vi "LSMcontroller_v64_updatedwaveformhandling.vi"() -> ()   [LabVIEW 2015] (continued)
                                n91 = local write "# of frames"(1 ("# of frames")) -> ()
                                }
                                }
                                }
                                }
                              }
                            }
                          }
                        }
                        n92 = local write "ROI Type"(w2086) -> ()
                      }
                      frame #1 {
                        # "change active waveform numbers array"
                        n93 = local read "save\ndata"() -> (w2126:bool)
                        n94 = Get Date/Time In Seconds() -> (seconds since 1Jan1904=w2128:timestamp)
                        n95 = case shown="True" w2126 {
                          tunnel: w2128 -> [w2129 w2131]
                          tunnel: [w2129 w2130] -> w2127
                          frame False {
                          }
                          frame True {
                            n96 = call "createdatafolder.vi"("timestamp in"=w2131) -> ("current data path"=w2132:path, "timestamp out"=w2130:timestamp)
                            n97 = local write "data dir"(w2132) -> ()
                          }
                        }
                        n98 = stacked-sequence {
                          tunnel: w2127 -> [_ w2139 _ _ _ _ _ _ _ _]
                          tunnel: [_ _ _ _ _ w2282 _ _ _ _] -> w2125
                          tunnel: [_ _ _ _ _ w2281 _ _ _ _] -> w2124
                          tunnel: [_ _ _ _ _ w2280 _ _ _ _] -> w2123
                          tunnel: [_ _ _ _ _ w2279 _ _ _ _] -> w2122
                          tunnel: [_ _ _ _ _ w2278 _ _ _ _] -> w2121
                          tunnel: [_ _ _ _ _ w2277 _ _ _ _] -> w2120
                          tunnel: [_ _ _ _ _ w2276 _ _ _ _] -> w2119
                          tunnel: [_ _ _ _ _ w2275 _ _ _ _] -> w2118
                          tunnel: [_ _ _ _ _ w2274 _ _ _ _] -> w2117
                          tunnel: [_ _ _ _ _ w2273 _ _ _ _] -> w2116
                          tunnel: [_ _ _ _ _ w2272 _ _ _ _] -> w2115
                          tunnel: [_ _ _ _ _ w2271 _ _ _ _] -> w2114
                          tunnel: [_ _ _ _ _ w2270 _ _ _ _] -> w2113
                          tunnel: [_ _ _ _ _ w2269 _ _ _ _] -> w2112
                          frame #0 {
                            n99 = local read "AI channels"() -> (w2138:i32[])
                            n100 = local read "CI channels"() -> (w2137:i32[])
                            n101 = call "2pparameters.vi"("command"="get") -> ("params out"=w2135:T10)  [unwired: 1 in]
                            n102 = Bundle By Name(cluster=w2135, "aAI"=w2138, "aCI"=w2137) -> (w2136:T10)
                            n103 = call "2pparameters.vi"("Params in"=w2136, "command"="set") -> ()  [unwired: 1 out]
                          }
                          frame #1 {
                            n104 = local read "Vy-min ref"() -> (w2143:dbl)
                            n105 = local read "Vy-max ref"() -> (w2144:dbl)
                            n106 = local read "Angle ref"() -> (w2142:dbl)
                            n107 = local read "Vx-min ref"() -> (w2145:dbl)
                            n108 = local write "counts"(0 ("counts")) -> ()
                            n109 = local write "graphtab"(T5."image" ("graphtab")) -> ()
                            n110 = local read "Vx-max ref"() -> (w2146:dbl)
                            n111 = property on="Stop" class="Bool (strict)"("Visible"=TRUE, "DisabledEnum"=T7."Enabled" ("Disabled")) -> ()  [unwired: 2 in, 2 out]
                            n112 = property on="Start" class="Bool (strict)"("Visible"=FALSE, "DisabledEnum"=T7."Disabled and Grayed Out" ("Disabled")) -> ()  [unwired: 2 in, 2 out]
                            n113 = script code="Xic=(ximax+ximin)./2;\nYic=(yimax+yimin)./2;\nximin=ximin-Xic;\nymin=ymin-Yic;\nxirmin=ximin.*cos(pi/180.*phi)+yimin.*sin(pi./180.*phi)+Xic;\nyirmin=-ximin.*sin(pi./180.*phi)+yimin.*cos(pi./180.*phi)+Yic;"("ximax"=w2146, "ximin"=w2145, "yimax"=w2144, "yimin"=w2143, "phi"=w2142) -> ("xirmin"=w2141:dbl, "yirmin"=w2140:dbl)  [unwired: 1 in, 1 out]
                            n114 = stacked-sequence {
                              tunnel: w2139 -> [_ w2171 _]
                              frame #0 {
                                n115 = local read "Measurement"() -> (w2153:T4)
                                n116 = case shown="\"X-Y-Z stack\"" w2153 {
                                frame "X-Y-t movie", Default {
                                n117 = call "2pparameters.vi"("command"="get") -> ("params out"=w2156:T10)  [unwired: 1 in]
                                n118 = Bundle By Name(cluster=w2156, "type"="X-Y-t movie") -> (w2154:T10)
                                n119 = call "2pparameters.vi"("Params in"=w2154, "command"="set") -> ()  [unwired: 1 out]
                                }
                                frame "X-Y-Z stack" {
                                n120 = call "2pparameters.vi"("command"="get") -> ("params out"=w2161:T10)  [unwired: 1 in]
                                n121 = Bundle By Name(cluster=w2161, "type"="X-Y-Z stack") -> (w2159:T10)
                                n122 = call "2pparameters.vi"("Params in"=w2159, "command"="set") -> ()  [unwired: 1 out]
                                }
                                frame "Lifetime (scan)" {
                                n123 = call "2pparameters.vi"("command"="get") -> ("params out"=w2166:T10)  [unwired: 1 in]
                                n124 = Bundle By Name(cluster=w2166, "type"="Lifetime (scan)") -> (w2164:T10)
                                n125 = call "2pparameters.vi"("Params in"=w2164, "command"="set") -> ()  [unwired: 1 out]
                                }
                                }
                              }
                              frame #1 {
                                n126 = Format Date/Time String(time format string (%c)="%Y%m%d", seconds (now)=w2171) -> (date/time string=w2170:string)  [unwired: 1 in]
                                n127 = Format Date/Time String(time format string (%c)="%H%M%S", seconds (now)=w2171) -> (date/time string=w2169:string)  [unwired: 1 in]
                                n128 = call "2pparameters.vi"("command"="get") -> ("params out"=w2175:T10)  [unwired: 1 in]
                                n129 = Bundle By Name(cluster=w2175, "date"=w2170, "time"=w2169) -> (w2174:T10)
                                n130 = call "2pparameters.vi"("Params in"=w2174, "command"="set") -> ()  [unwired: 1 out]
                              }
                              frame #2 {
                                n131 = call "configuration.vi"("command"="get") -> ("config out"=w2185:T11)  [unwired: 2 in, 1 out]
                                n132 = Unbundle By Name(w2185) -> ("CI names"=w2186:string[], "AI names"=w2187:string[])
                                n133 = call "2pparameters.vi"("command"="get") -> ("params out"=w2181:T10)  [unwired: 1 in]
                                n134 = Unbundle By Name(w2181) -> ("aCI"=w2182:i32[], "aAI"=w2183:i32[])
                                n135 = for {
                                tunnel: w2182 -> [w2197] mode=indexing
                                tunnel: w2186 -> [w2198]
                                tunnel: [w2196] -> w2188 mode=indexing
                                n136 = Index Array(array=w2198, index=w2197) -> (element=w2196:string)
                                }
                                n137 = for {
                                tunnel: w2183 -> [w2194] mode=indexing
                                tunnel: w2187 -> [w2195]
                                tunnel: [w2193] -> w2189 mode=indexing
                                n138 = Index Array(array=w2195, index=w2194) -> (element=w2193:string)
                                }
                                n139 = Build Array (concatenate)(w2188, w2189) -> (w2179:string[])
                                n140 = for {
                                tunnel: w2179 -> [w2191] mode=indexing
                                tunnel: [w2190] -> w2178 mode=indexing
                                i -> [w2192]
                                n141 = Bundle("String"=w2191, w2192) -> (w2190:cluster{"String":string, i32})  [unwired: 1 in]
                                }
                                n142 = property on="image1list" class="Ring (strict)"("StringsAndValues[]"=w2178) -> ()  [unwired: 2 in, 2 out]
                                n143 = property on="image2list" class="Ring (strict)"("StringsAndValues[]"=w2178) -> ()  [unwired: 2 in, 2 out]
                              }
                            }
                            n144 = call "setposition.vi"("Vy"=w2140, "Vx"=w2141) -> ()  [unwired: 1 in]
                          }
                          frame #2 {
                            n145 = call "X-array-databuffer.vi"("command"=enum16{"get", "set", "clear", "append"}."clear") -> ()  [unwired: 3 in, 2 out]
                            n146 = call "Y-array-databuffer.vi"("command"=enum16{"get", "set", "clear", "append"}."clear") -> ()  [unwired: 3 in, 2 out]
                            n147 = call "2pparameters.vi"("command"="get") -> ("params out"=w2201:T10)  [unwired: 1 in]
                            n148 = Unbundle By Name(w2201) -> ("autoshutter"=w2202:bool, "auto OD"=w2199:bool)
                            n149 = call "allAI-temp_img.vi"("command"=enum16{"get", "set", "clear", "append"}."clear") -> ()  [unwired: 3 in, 2 out]
                            n150 = case shown="True" w2199 {
                              frame False {
                              }
                              frame True {
                                n151 = call "configuration.vi"("command"="get") -> ("config out"=w2210:T11)  [unwired: 2 in, 1 out]
                                n152 = Unbundle By Name(w2210) -> ("image OD"=w2211:u16)
                                n153 = local read "ODfilt"() -> (w2208:u16)
                                n154 = call "filterwheelcontrol_nothorlabslib.vi"("Current OD filt"=w2208, "New ODfilt"=w2211) -> ()  [unwired: 1 in]
                              }
                            }
                            n155 = case shown="True" w2202 {
                              frame False {
                              }
                              frame True {
                                n156 = call "shuttercontrol.vi"("command"="close") -> ()  [unwired: 1 in, 1 out]
                              }
                            }
                            n157 = call "CH1-temp.vi"("command"=enum16{"get", "set", "clear", "add row"}."clear") -> ()  [unwired: 3 in, 2 out]
                            n158 = call "CH2-temp.vi"("command"=enum16{"get", "set", "clear", "add row"}."clear") -> ()  [unwired: 3 in, 2 out]
                          }
                          frame #3 {
                            n159 = local read "avpp"() -> (w2245:i32)
                            n160 = local read "Angle ref"() -> (w2244:dbl)
                            n161 = local read "ROI Type"() -> (w2243:u16)
                            n162 = local read "xpixels ref"() -> (w2240:i32)
                            n163 = local read "Vx-min ref"() -> (w2239:dbl)
                            n164 = local read "Vx-max ref"() -> (w2238:dbl)
                            n165 = local read "ypixels ref"() -> (w2236:i32)
                            n166 = local read "Vy-min ref"() -> (w2237:dbl)
                            n167 = local read "Vy-max ref"() -> (w2233:dbl)
                            n168 = local read "Sampling rate"() -> (w2227:dbl)
                            n169 = local read "finite samples"() -> (w2228:bool)
                            n170 = local read "continuous"() -> (w2231:bool)
                            n171 = local read "wavdet"() -> (w2232:bool)
                            n172 = local read "# of frames"() -> (w2230:i32)
                            n173 = local read "maxbufferAI"() -> (w2229:i32)
                            n174 = local read "Override AI buffer"() -> (w2213:bool)
                            n175 = call "2pparameters.vi"("command"="get") -> ("params out"=w2242:T10)  [unwired: 1 in]
                            n176 = Bundle By Name(cluster=w2242, "avpp"=w2245, "Angle Img"=w2244, "Xpixels Img"=w2240, "Vx-min Img"=w2239, "VX-max Img"=w2238, "Ypixels Img"=w2236, "Vy-min Img"=w2237, "Vy-max Img"=w2233, "srate"=w2227, "srate Img"=w2227, "finite"=w2228, "cont"=w2231, "wavdet"=w2232, "measpoints"=w2230, "maxbufferAI"=w2229, "Drawing Mode"=w2243, "Vz-reset"=0.0, "AIoverride"=w2213) -> (w2234:T10)
                            n177 = call "2pparameters.vi"("Params in"=w2234, "command"="set") -> ()  [unwired: 1 out]
                            n178 = local read "Vholding (mV)"() -> (w2216:sgl)
                            n179 = local read "Current Clamp"() -> (w2222:bool)
                            n180 = local read "Voltage Clamp"() -> (w2221:bool)
                            n181 = local read "OCgain"() -> (w2217:sgl)
                            n182 = local read "CC_ICgain"() -> (w2220:dbl)
                            n183 = local read "holdon"() -> (w2215:bool)
                            n184 = call "patchparameters.vi"("command"="get") -> ("Params out"=w2224:T13)  [unwired: 1 in]
                            n185 = Bundle By Name(cluster=w2224, "VC"=w2221, "CC"=w2222, "CC_icg (pA/mv)"=w2220, "VC_icg (mV/mV)"=sgl 10.0, "OCG (mV/pA)"=w2217, "OVG (mV/mV)"=0.1, "Vhold (mV)"=w2216, "holdon"=w2215) -> (w2223:T13)
                            n186 = call "patchparameters.vi"("Params in"=w2223, "command"="set") -> ()  [unwired: 1 out]
                          }
                          frame #4 {
                            # "Generate Waveforms for Scanning Mirrors"
                            n187 = call "2pparameters.vi"("command"="get") -> ("params out"=w2260:T10)  [unwired: 1 in]
                            n188 = Unbundle By Name(w2260) -> ("srate Img"=w2259:sgl, "Angle Img"=w2258:dbl, "VX-max Img"=w2257:dbl, "Vx-min Img"=w2256:dbl, "Xpixels Img"=w2255:i32, "Ypixels Img"=w2254:i32, "Vy-max Img"=w2253:dbl, "Vy-min Img"=w2252:dbl, "Drawing Mode"=w2251:u16)
                            n189 = call "ROI-databuffer.vi"("command"=enum16{"get", "set", "clear", "append"}."get") -> ("array out"=w2250:cluster{"x":sgl, "y":sgl}[])  [unwired: 4 in]
                            n190 = call "ScanningWaveform_v4.vi"("Vy-min"=w2252, "Vy-max"=w2253, "yPixels/tPixels"=w2254, "xPixels/rPixels"=w2255, "Vx-min"=w2256, "Vx-max"=w2257, "Drawing Mode"=w2251, "Angle"=w2258, "AOrate"=w2259, "Points"=w2250) -> ("numPixels"=w2246:dbl, "Y-WaveArray"=w2249:dbl[], "P"=w2247:dbl, "X-WaveArray"=w2248:dbl[])  [unwired: 6 in]
                            n191 = call "2pparameters.vi"("command"="get") -> ("params out"=w2268:T10)  [unwired: 1 in]
                            n192 = call "Y-array-databuffer.vi"("array in"=w2249, "command"=enum16{"get", "set", "clear", "append"}."set") -> ()  [unwired: 2 in, 2 out]
                            n193 = call "X-array-databuffer.vi"("array in"=w2248, "command"=enum16{"get", "set", "clear", "append"}."set") -> ()  [unwired: 2 in, 2 out]
                            n194 = Bundle By Name(cluster=w2268, "P"=w2247, "sAOxy"=w2246) -> (w2265:T10)
                            n195 = call "2pparameters.vi"("Params in"=w2265, "command"="set") -> ()  [unwired: 1 out]
                          }
                          frame #5 {
                            # "rem2Ps"
                            # "A2Ps"
                            # "Al"
                            # "Rl"
                            n196 = stacked-sequence {
                              seq-local: [w2287 _ _ _ _ _ _ _ _ _ _] -> [_ w2399 _ w2454 _ w2534 _ _ _ _ _]
                              seq-local: [w2288 _ _ _ _ _ _ _ _ _ _] -> [_ w2400 w2410 _ w2503 _ _ _ _ _ _]
                              seq-local: [_ _ w2409 _ _ _ _ _ _ _ _] -> [_ _ _ _ w2497 _ _ _ _ _ _]
                              seq-local: [_ _ _ w2453 _ _ _ _ _ _ _] -> [_ _ _ _ _ w2533 _ _ _ _ _]
                              seq-local: [w2284 _ _ _ _ _ _ _ _ _ _] -> [_ w2396 _ _ _ _ _ _ w2719 w2787 _]
                              seq-local: [w2283 _ _ _ _ _ _ _ _ _ _] -> [_ w2395 _ _ _ _ _ _ w2720 w2788 _]
                              seq-local: [w2290 _ _ _ _ _ _ _ _ _ _] -> [_ _ _ _ _ _ w2572 _ w2718 w2786 _]
                              seq-local: [w2286 _ _ _ _ _ _ _ _ _ _] -> [_ w2394 _ _ _ _ w2571 w2639 _ _ _]
                              seq-local: [w2285 _ _ _ _ _ _ _ _ _ _] -> [_ w2393 _ _ _ _ w2570 w2638 _ _ _]
                              seq-local: [w2289 _ _ _ _ _ _ _ _ _ _] -> [_ _ _ _ _ _ w2569 w2637 _ _ _]
                              tunnel: [_ _ w2408 _ _ _ _ _ _ _ _] -> w2281
                              tunnel: [_ _ w2407 _ _ _ _ _ _ _ _] -> w2280
                              tunnel: [w2288 _ _ _ _ _ _ _ _ _ _] -> w2282
                              tunnel: [w2287 _ _ _ _ _ _ _ _ _ _] -> w2279
                              tunnel: [_ _ _ w2452 _ _ _ _ _ _ _] -> w2278
                              tunnel: [_ _ _ w2451 _ _ _ _ _ _ _] -> w2277
                              tunnel: [w2286 _ _ _ _ _ _ _ _ _ _] -> w2276
                              tunnel: [w2285 _ _ _ _ _ _ _ _ _ _] -> w2275
                              tunnel: [_ _ _ _ _ _ w2568 _ _ _ _] -> w2274
                              tunnel: [_ _ _ _ _ _ _ w2636 _ _ _] -> w2273
                              tunnel: [w2284 _ _ _ _ _ _ _ _ _ _] -> w2272
                              tunnel: [w2283 _ _ _ _ _ _ _ _ _ _] -> w2271
                              tunnel: [_ _ _ _ _ _ _ _ w2717 _ _] -> w2270
                              tunnel: [_ _ _ _ _ _ _ _ _ w2785 _] -> w2269
                              frame #0 {
                                # "for a next version, give ome thought to\nthe possibilit of intermittently updating the\nwaveforms. it will have to be a calculation\nbased on speed of CPU and program on the one hand\nand length of measurement on the other. but then it should be possible, in principle, to \nupdate the waveform on the fly and that way cut up a longer measurement in smaller parts."
                                # "Y"
                                # "X"
                                n197 = stacked-sequence {
                                tunnel: [w2291 _ _ _] -> w2288
                                tunnel: [_ w2303 _ _] -> w2287
                                tunnel: [_ _ _ w2360] -> w2283
                                tunnel: [_ _ _ w2359] -> w2284
                                tunnel: [_ _ _ w2358] -> w2290
                                tunnel: [_ _ w2318 _] -> w2286
                                tunnel: [_ _ w2317 _] -> w2285
                                tunnel: [_ _ w2316 _] -> w2289
                                frame #0 {
                                n198 = call "configuration.vi"("command"="get") -> ("config out"=w2293:T11)  [unwired: 2 in, 1 out]
                                n199 = Unbundle By Name(w2293) -> ("Voltage to Xgalvo"=w2292:i32)
                                n200 = call "2pparameters.vi"("command"="get") -> ("params out"=w2297:T10)  [unwired: 1 in]
                                n201 = in-place {
                                in-place-border: w2292 -> [w2302]
                                in-place-border: [w2299] -> w2291
                                n202 = in-place-cluster #1(w2297) -> ("aAO"=w2301:u32[])
                                n203 = call "add channel to active arrayv2.vi"("line array in"=w2301, "line to add"=w2302) -> ("line array out"=w2300:u32[], "addition"=w2299:bool)  [unwired: 1 out]
                                n204 = in-place-cluster #1("aAO"=w2300) -> (w2295:T10)
                                }
                                n205 = call "2pparameters.vi"("Params in"=w2295, "command"="set") -> ()  [unwired: 1 out]
                                }
                                frame #1 {
                                n206 = call "configuration.vi"("command"="get") -> ("config out"=w2305:T11)  [unwired: 2 in, 1 out]
                                n207 = Unbundle By Name(w2305) -> ("Voltage to Ygalvo"=w2304:i32)
                                n208 = call "2pparameters.vi"("command"="get") -> ("params out"=w2309:T10)  [unwired: 1 in]
                                n209 = in-place {
                                in-place-border: w2304 -> [w2314]
                                in-place-border: [w2311] -> w2303
                                n210 = in-place-cluster #2(w2309) -> ("aAO"=w2313:u32[])
                                n211 = call "add channel to active arrayv2.vi"("line array in"=w2313, "line to add"=w2314) -> ("line array out"=w2312:u32[], "addition"=w2311:bool)  [unwired: 1 out]
                                n212 = in-place-cluster #2("aAO"=w2312) -> (w2307:T10)
                                }
                                n213 = call "2pparameters.vi"("Params in"=w2307, "command"="set") -> ()  [unwired: 1 out]
                                }
                                frame #2 {
                                n214 = call "2pparameters.vi"("command"="get") -> ("params out"=w2320:T10)  [unwired: 1 in]
                                n215 = Unbundle By Name(w2320) -> ("autoshutter"=w2319:bool, "wavdet"=w2315:bool)
                                n216 = case shown="True" w2319 {
                                tunnel: [w2325 w2345] -> w2318
                                tunnel: [w2324 FALSE ("removal")] -> w2317
                                tunnel: [w2323 w2343] -> w2316
                                tunnel: w2315 -> [w2322 _]
                                frame False {
                                n217 = case shown="False" w2322 {
                                tunnel: [FALSE ("addition") FALSE ("addition")] -> w2325
                                tunnel: [w2327 FALSE ("removal")] -> w2324
                                tunnel: [w2326 _] -> w2323
                                frame False {
                                n218 = call "configuration.vi"("command"="get") -> ("config out"=w2333:T11)  [unwired: 2 in, 1 out]
                                n219 = Unbundle By Name(w2333) -> ("2P shutter"=w2330:i32)
                                n220 = call "2pparameters.vi"("command"="get") -> ("params out"=w2331:T10)  [unwired: 1 in]
                                n221 = in-place {
                                in-place-border: w2330 -> [w2340]
                                in-place-border: [w2337] -> w2327
                                in-place-border: [w2336] -> w2326
                                n222 = in-place-cluster #3(w2331) -> ("aDO"=w2339:u32[])
                                n223 = call "remove channel from active arrayv2.vi"("line array in"=w2339, "line to remove"=w2340) -> ("line array out"=w2338:u32[], "removal"=w2337:bool, "index"=w2336:i32)
                                n224 = in-place-cluster #3("aDO"=w2338) -> (w2328:T10)
                                }
                                n225 = call "2pparameters.vi"("Params in"=w2328, "command"="set") -> ()  [unwired: 1 out]
                                }
                                frame True {
                                }
                                }
                                }
                                frame True {
                                n226 = call "configuration.vi"("command"="get") -> ("config out"=w2347:T11)  [unwired: 2 in, 1 out]
                                n227 = call "2pparameters.vi"("command"="get") -> ("params out"=w2351:T10)  [unwired: 1 in]
                                n228 = Unbundle By Name(w2347) -> ("2P shutter"=w2346:i32)
                                n229 = in-place {
                                in-place-border: w2346 -> [w2357]
                                in-place-border: [w2354] -> w2345
                                in-place-border: [w2353] -> w2343
                                n230 = in-place-cluster #4(w2351) -> ("aDO"=w2356:u32[])
                                n231 = call "add channel to active arrayv2.vi"("line array in"=w2356, "line to add"=w2357) -> ("line array out"=w2355:u32[], "addition"=w2354:bool, "index"=w2353:i32)
                                n232 = in-place-cluster #4("aDO"=w2355) -> (w2349:T10)
                                }
                                n233 = call "2pparameters.vi"("Params in"=w2349, "command"="set") -> ()  [unwired: 1 out]
                                }
                                }
                                }
                                frame #3 {
                                n234 = local read "Measurement"() -> (w2361:T4)
                                n235 = To Unsigned Long Integer(number=w2361) -> (unsigned 32bit integer=w2362:u32)
                                n236 = case shown="5..7" w2362 {
                                tunnel: [FALSE ("addition") w2380] -> w2360
                                tunnel: [w2365 FALSE ("removal")] -> w2359
                                tunnel: [w2363 w2378] -> w2358
                                frame 0..4, Default {
                                n237 = call "configuration.vi"("command"="get") -> ("config out"=w2371:T11)  [unwired: 2 in, 1 out]
                                n238 = Unbundle By Name(w2371) -> ("LT timestamp"=w2368:u32)
                                n239 = call "2pparameters.vi"("command"="get") -> ("params out"=w2369:T10)  [unwired: 1 in]
                                n240 = in-place {
                                in-place-border: w2368 -> [w2377]
                                in-place-border: [w2374] -> w2365
                                in-place-border: [w2373] -> w2363
                                n241 = in-place-cluster #5(w2369) -> ("aDO"=w2376:u32[])
                                n242 = call "remove channel from active arrayv2.vi"("line array in"=w2376, "line to remove"=w2377) -> ("line array out"=w2375:u32[], "removal"=w2374:bool, "index"=w2373:i32)
                                n243 = in-place-cluster #5("aDO"=w2375) -> (w2366:T10)
                                }
                                n244 = call "2pparameters.vi"("Params in"=w2366, "command"="set") -> ()  [unwired: 1 out]
                                }
                                frame 5..7 {
                                n245 = call "configuration.vi"("command"="get") -> ("config out"=w2386:T11)  [unwired: 2 in, 1 out]
                                n246 = Unbundle By Name(w2386) -> ("LT timestamp"=w2383:u32)
                                n247 = call "2pparameters.vi"("command"="get") -> ("params out"=w2384:T10)  [unwired: 1 in]
                                n248 = in-place {
                                in-place-border: w2383 -> [w2392]
                                in-place-border: [w2389] -> w2380
                                in-place-border: [w2388] -> w2378
                                n249 = in-place-cluster #6(w2384) -> ("aDO"=w2391:u32[])
                                n250 = call "add channel to active arrayv2.vi"("line array in"=w2391, "line to add"=w2392) -> ("line array out"=w2390:u32[], "addition"=w2389:bool, "index"=w2388:i32)
                                n251 = in-place-cluster #6("aDO"=w2390) -> (w2381:T10)
                                }
                                n252 = call "2pparameters.vi"("Params in"=w2381, "command"="set") -> ()  [unwired: 1 out]
                                }
                                }
                                }
                                }
                              }
                              frame #1 {
                                n253 = Or(x=w2399, y=w2400) -> (x .or. y?=w2398:bool)
                                n254 = case shown="True" w2398 {
                                frame False {
                                }
                                frame True {
                                # "update GUI"
                                n255 = call "Used AO lines.vi"() -> ("used AO names"=w2404:string[], "used AO lines"=w2406:tag[])  [unwired: 2 in]
                                n256 = control-ref of="Analog Lines Plot"() -> (w2405:refnum<vi>)
                                n257 = local write "Analog Used Lines"(w2406) -> ()
                                n258 = local write "Analog Used Names"(w2404) -> ()
                                n259 = call "prepAOWaveplot.vi"("WaveformGraph in"=w2405, "Analog Used Names"=w2404) -> ()  [unwired: 1 in]
                                }
                                }
                                n260 = Compound Arithmetic op=OR(w2396, w2395, w2394, w2393) -> (w2397:bool)
                                n261 = case shown="True" w2397 {
                                frame False {
                                }
                                frame True {
                                n262 = control-ref of="Digital Lines Plot"() -> (w2401:refnum<vi>)
                                n263 = call "Used DO lines.vi"() -> ("used DO names"=w2402:string[], "used DO lines"=w2403:tag[])  [unwired: 2 in]
                                n264 = local write "Digital Used Lines"(w2403) -> ()
                                n265 = local write "Digital Used Names"(w2402) -> ()
                                n266 = call "prepDOWaveplot.vi"("DigitalGraph in"=w2401, "used DO names"=w2402) -> ()  [unwired: 1 in]
                                }
                                }
                              }
                              frame #2 {
                                n267 = case shown="False" w2410 {
                                tunnel: [w2413 w2434] -> w2409
                                tunnel: [w2412 w2432] -> w2408
                                tunnel: [w2411 _] -> w2407
                                frame False {
                                n268 = stacked-sequence {
                                seq-local: [w2415 _] -> [_ w2428]
                                tunnel: [w2415 _] -> w2413
                                tunnel: [w2418 _] -> w2412
                                tunnel: [w2414 _] -> w2411
                                frame #0 {
                                n269 = call "configuration.vi"("command"="get") -> ("config out"=w2426:T11)  [unwired: 2 in, 1 out]
                                n270 = call "waveformparamsv2.vi"("command"="get") -> ("Params out"=w2420:T14)  [unwired: 4 in, 2 out]
                                n271 = Unbundle By Name(w2426) -> ("Voltage to Xgalvo"=w2427:i32)
                                n272 = call "2pparameters.vi"("command"="get") -> ("params out"=w2423:T10)  [unwired: 1 in]
                                n273 = Unbundle By Name(w2420) -> ("AO parameters"=w2419:T15)
                                n274 = Unbundle By Name(w2423) -> ("aAO"=w2424:u32[])
                                n275 = call "waveformsAObuffer.vi"("command"="get") -> ("AO wf out"=w2416:waveform(dbl)[])  [unwired: 1 in]
                                n276 = Search 1D Array(1D array=w2424, element=w2427) -> (index of element=w2415:i32)  [unwired: 1 in]
                                n277 = Index Array(array=w2416, index=w2415) -> (element=w2414:waveform(dbl))
                                n278 = Index Array(array=w2419, index=w2415) -> (element=w2418:T16)
                                }
                                frame #1 {
                                w2429 = 0.0 ("Step size (V)")
                                n279 = local read "Sampling rate"() -> (w2430:dbl)
                                n280 = call "replace AO XYwfparam.vi"("Baseline (V)"=w2429, "Start amplitude (V)"=w2429, "Cycles"=w2429, "Repeats"=w2429, "index of AO wave"=w2428, "Step size (V)"=w2429, "DC (%)"=w2429, "Sampling frequency (Hz)"=w2430, "Period (ms)"=w2429, "Cycle length (s)"=w2429, "Pulses"=w2429, "padding value"=w2429, "Matlab wave name"=path "xwave") -> ()  [unwired: 3 in]
                                }
                                }
                                }
                                frame True {
                                w2433 = 0.0 ("Repeats")
                                n281 = local read "Sampling rate"() -> (w2442:dbl)
                                n282 = call "2pparameters.vi"("command"="get") -> ("params out"=w2436:T10)  [unwired: 1 in]
                                n283 = call "configuration.vi"("command"="get") -> ("config out"=w2439:T11)  [unwired: 2 in, 1 out]
                                n284 = call "waveformparamsv2.vi"("command"="get") -> ("Params out"=w2448:T14)  [unwired: 4 in, 2 out]
                                n285 = Unbundle By Name(w2439) -> ("Voltage to Xgalvo"=w2440:i32)
                                n286 = Unbundle By Name(w2448) -> ("AO parameters"=w2445:T15)
                                n287 = Unbundle By Name(w2436) -> ("aAO"=w2437:u32[])
                                n288 = Search 1D Array(1D array=w2437, element=w2440) -> (index of element=w2434:i32)  [unwired: 1 in]
                                n289 = Index Array(array=w2445, index=0) -> (element=w2446:T16)
                                n290 = Bundle By Name(cluster=w2446, "AOtab"=-1.0 ("Repeats"), "Repeats"=w2433, "Cycles"=w2433, "Start amplitude (V)"=w2433, "Baseline (V)"=w2433, "Step size (V)"=w2433, "DC (%)"=w2433, "Sampling frequency (Hz)"=w2442, "Period (ms)"=w2433, "Offset (V)"=w2433, "Amplitude (V)"=w2433, "Frequency"=w2433, "Tri Repeats"=w2433, "phase shift (ms)"=w2433, "Pulses"=w2433, "Matlab wave file"=path "xwave", "padding value"=w2433) -> (w2432:T16)
                                n291 = Build Array(w2432) -> (w2443:T15)
                                n292 = call "waveformparamsv2.vi"("command"="add AO", "add AO"=w2443) -> ()  [unwired: 3 in, 3 out]
                                }
                                }
                              }
                              frame #3 {
                                n293 = case shown="False" w2454 {
                                tunnel: [w2457 w2478] -> w2453
                                tunnel: [w2456 w2476] -> w2452
                                tunnel: [w2455 _] -> w2451
                                frame False {
                                n294 = stacked-sequence {
                                seq-local: [w2459 _] -> [_ w2472]
                                tunnel: [w2459 _] -> w2457
                                tunnel: [w2462 _] -> w2456
                                tunnel: [w2458 _] -> w2455
                                frame #0 {
                                n295 = call "configuration.vi"("command"="get") -> ("config out"=w2470:T11)  [unwired: 2 in, 1 out]
                                n296 = call "waveformparamsv2.vi"("command"="get") -> ("Params out"=w2464:T14)  [unwired: 4 in, 2 out]
                                n297 = Unbundle By Name(w2470) -> ("Voltage to Ygalvo"=w2471:i32)
                                n298 = call "2pparameters.vi"("command"="get") -> ("params out"=w2467:T10)  [unwired: 1 in]
                                n299 = Unbundle By Name(w2464) -> ("AO parameters"=w2463:T15)
                                n300 = Unbundle By Name(w2467) -> ("aAO"=w2468:u32[])
                                n301 = call "waveformsAObuffer.vi"("command"="get") -> ("AO wf out"=w2460:waveform(dbl)[])  [unwired: 1 in]
                                n302 = Search 1D Array(1D array=w2468, element=w2471) -> (index of element=w2459:i32)  [unwired: 1 in]
                                n303 = Index Array(array=w2460, index=w2459) -> (element=w2458:waveform(dbl))
                                n304 = Index Array(array=w2463, index=w2459) -> (element=w2462:T16)
                                }
                                frame #1 {
                                w2473 = 0.0 ("Step size (V)")
                                n305 = local read "Sampling rate"() -> (w2474:dbl)
                                n306 = call "replace AO XYwfparam.vi"("Baseline (V)"=w2473, "Start amplitude (V)"=w2473, "Cycles"=w2473, "Repeats"=w2473, "index of AO wave"=w2472, "Step size (V)"=w2473, "DC (%)"=w2473, "Sampling frequency (Hz)"=w2474, "Period (ms)"=w2473, "Cycle length (s)"=w2473, "Pulses"=w2473, "padding value"=w2473, "Matlab wave name"=path "ywave") -> ()  [unwired: 3 in]
                                }
                                }
                                }
                                frame True {
                                w2477 = 0.0 ("Repeats")
                                n307 = local read "Sampling rate"() -> (w2487:dbl)
                                n308 = call "2pparameters.vi"("command"="get") -> ("params out"=w2480:T10)  [unwired: 1 in]
                                n309 = call "configuration.vi"("command"="get") -> ("config out"=w2483:T11)  [unwired: 2 in, 1 out]
                                n310 = call "waveformparamsv2.vi"("command"="get") -> ("Params out"=w2493:T14)  [unwired: 4 in, 2 out]
                                n311 = Unbundle By Name(w2483) -> ("Voltage to Ygalvo"=w2484:i32)
                                n312 = Unbundle By Name(w2493) -> ("AO parameters"=w2490:T15)
                                n313 = Unbundle By Name(w2480) -> ("aAO"=w2481:u32[])
                                n314 = Search 1D Array(1D array=w2481, element=w2484) -> (index of element=w2478:i32)  [unwired: 1 in]
                                n315 = Index Array(array=w2490, index=0) -> (element=w2491:T16)
                                n316 = Bundle By Name(cluster=w2491, "AOtab"=-1.0 ("Repeats"), "Repeats"=w2477, "Cycles"=w2477, "Start amplitude (V)"=w2477, "Baseline (V)"=w2477, "Step size (V)"=w2477, "DC (%)"=w2477, "Sampling frequency (Hz)"=w2487, "Period (ms)"=w2477, "Offset (V)"=w2477, "Amplitude (V)"=w2477, "Frequency"=w2477, "Tri Repeats"=w2477, "phase shift (ms)"=w2477, "Pulses"=w2477, "Matlab wave file"=path "ywave", "padding value"=w2477) -> (w2476:T16)
                                n317 = Build Array(w2476) -> (w2488:T15)
                                n318 = call "waveformparamsv2.vi"("command"="add AO", "add AO"=w2488) -> ()  [unwired: 3 in, 3 out]
                                }
                                }
                              }
                              frame #4 {
                                n319 = call "2pparameters.vi"("command"="get") -> ("params out"=w2500:T10)  [unwired: 1 in]
                                n320 = Unbundle By Name(w2500) -> ("wavdet"=w2499:bool, "sAOxy"=w2496:i32, "refwfsize"=w2495:dbl, "srate Img"=w2498:sgl)
                                n321 = case shown="False" w2499 {
                                tunnel: [w2504 w2514] -> w2502
                                tunnel: w2498 -> [w2505 w2516]
                                tunnel: w2496 -> [_ w2512]
                                tunnel: w2495 -> [_ w2511]
                                frame False {
                                n322 = call "X-array-databuffer.vi"("command"=enum16{"get", "set", "clear", "append"}."get") -> ("array out"=w2508:dbl[])  [unwired: 3 in, 1 out]
                                n323 = Reciprocal(x=w2505) -> (1/x=w2506:sgl)
                                n324 = Bundle By Name("Y"=w2508, "dt"=w2506) -> (w2504:waveform(dbl))  [unwired: 1 in]
                                }
                                frame True {
                                n325 = To Double Precision Float(number=w2512) -> (double precision float=w2513:dbl)
                                n326 = Divide(x=w2511, y=w2513) -> (x/y=w2509:dbl)
                                n327 = Round Toward +Infinity(x=w2509) -> (ceil(x): smallest int >= x=w2510:dbl)
                                n328 = call "X-array-databuffer.vi"("command"=enum16{"get", "set", "clear", "append"}."get") -> ("array out"=w2518:dbl[])  [unwired: 3 in, 1 out]
                                n329 = Reciprocal(x=w2516) -> (1/x=w2517:sgl)
                                n330 = for {
                                N: w2510 -> [_]
                                tunnel: w2518 -> [w2520]
                                tunnel: [w2520] -> w2515 mode=concatenating
                                }
                                n331 = Bundle By Name("Y"=w2515, "dt"=w2517) -> (w2514:waveform(dbl))  [unwired: 1 in]
                                }
                                }
                                n332 = case shown="False" w2503 {
                                tunnel: w2502 -> [w2522 w2528]
                                tunnel: w2497 -> [w2523 _]
                                frame False {
                                n333 = call "waveformsAObuffer.vi"("command"="get") -> ("AO wf out"=w2526:waveform(dbl)[])  [unwired: 1 in]
                                n334 = Replace Array Subset(array=w2526, new element=w2522, index=w2523) -> (w2521:waveform(dbl)[])
                                n335 = call "waveformsAObuffer.vi"("AO wf in"=w2521, "command"="set") -> ()  [unwired: 1 out]
                                }
                                frame True {
                                n336 = call "waveformsAObuffer.vi"("command"="get") -> ("AO wf out"=w2530:waveform(dbl)[])  [unwired: 1 in]
                                n337 = Build Array (concatenate)(w2530, w2528) -> (w2527:waveform(dbl)[])
                                n338 = call "waveformsAObuffer.vi"("AO wf in"=w2527, "command"="set") -> ()  [unwired: 1 out]
                                }
                                }
                              }
                              frame #5 {
                                n339 = call "2pparameters.vi"("command"="get") -> ("params out"=w2542:T10)  [unwired: 1 in]
                                n340 = Unbundle By Name(w2542) -> ("wavdet"=w2541:bool, "sAOxy"=w2539:i32, "refwfsize"=w2540:dbl, "srate Img"=w2535:sgl)
                                n341 = To Double Precision Float(number=w2539) -> (double precision float=w2538:dbl)
                                n342 = Divide(x=w2540, y=w2538) -> (x/y=w2537:dbl)
                                n343 = Round Toward +Infinity(x=w2537) -> (ceil(x): smallest int >= x=w2536:dbl)
                                n344 = case shown="True" w2541 {
                                tunnel: [w2546 w2551] -> w2532
                                tunnel: w2536 -> [_ w2555]
                                tunnel: w2535 -> [w2547 w2553]
                                frame False {
                                n345 = call "Y-array-databuffer.vi"("command"=enum16{"get", "set", "clear", "append"}."get") -> ("array out"=w2544:dbl[])  [unwired: 3 in, 1 out]
                                n346 = Reciprocal(x=w2547) -> (1/x=w2548:sgl)
                                n347 = Bundle By Name("Y"=w2544, "dt"=w2548) -> (w2546:waveform(dbl))  [unwired: 1 in]
                                }
                                frame True {
                                n348 = call "Y-array-databuffer.vi"("command"=enum16{"get", "set", "clear", "append"}."get") -> ("array out"=w2549:dbl[])  [unwired: 3 in, 1 out]
                                n349 = Reciprocal(x=w2553) -> (1/x=w2554:sgl)
                                n350 = for {
                                N: w2555 -> [_]
                                tunnel: w2549 -> [w2556]
                                tunnel: [w2556] -> w2552 mode=concatenating
                                }
                                n351 = Bundle By Name("Y"=w2552, "dt"=w2554) -> (w2551:waveform(dbl))  [unwired: 1 in]
                                }
                                }
                                n352 = case shown="False" w2534 {
                                tunnel: w2532 -> [w2559 w2564]
                                tunnel: w2533 -> [w2560 _]
                                frame False {
                                n353 = call "waveformsAObuffer.vi"("command"="get") -> ("AO wf out"=w2562:waveform(dbl)[])  [unwired: 1 in]
                                n354 = Replace Array Subset(array=w2562, new element=w2559, index=w2560) -> (w2557:waveform(dbl)[])
                                n355 = call "waveformsAObuffer.vi"("AO wf in"=w2557, "command"="set") -> ()  [unwired: 1 out]
                                }
                                frame True {
                                n356 = call "waveformsAObuffer.vi"("command"="get") -> ("AO wf out"=w2566:waveform(dbl)[])  [unwired: 1 in]
                                n357 = Build Array (concatenate)(w2566, w2564) -> (w2563:waveform(dbl)[])
                                n358 = call "waveformsAObuffer.vi"("AO wf in"=w2563, "command"="set") -> ()  [unwired: 1 out]
                                }
                                }
                              }
                              frame #6 {
                                n359 = Build Array(w2571, w2570) -> (w2574:bool[])
                                n360 = Boolean Array To Number(Boolean array=w2574) -> (number=w2573:u32)
                                n361 = case shown="0" w2573 {
                                tunnel: w2572 -> [_ _ _ _]
                                tunnel: w2569 -> [_ w2597 _ w2610]
                                tunnel: [_ w2596 _ w2607] -> w2568
                                frame 1 {
                                w2584 = 0.0 ("DOtab")
                                n362 = call "2pparameters.vi"("command"="get") -> ("params out"=w2581:T10)  [unwired: 1 in]
                                n363 = call "waveformparamsv2.vi"("command"="get") -> ("Params out"=w2592:T14)  [unwired: 4 in, 2 out]
                                n364 = Unbundle By Name(w2592) -> ("DO parameters"=w2590:T17)
                                n365 = Unbundle By Name(w2581) -> ("srate"=w2577:sgl, "sAOxy"=w2580:i32)
                                n366 = To Double Precision Float(number=w2577) -> (double precision float=w2575:dbl)
                                n367 = To Double Precision Float(number=w2577) -> (double precision float=w2576:dbl)
                                n368 = To Double Precision Float(number=w2580) -> (double precision float=w2579:dbl)
                                n369 = Divide(x=w2576, y=w2579) -> (x/y=w2578:dbl)
                                n370 = Index Array(array=w2590, index=0) -> (element=w2589:T18)
                                n371 = Bundle By Name(cluster=w2589, "Digital DC (%)"=100.0, "Digital phase"=w2584, "Digital Freq (Hz)"=w2578, "Sampling frequency (Hz)"=w2575, "Digital time offset (s)"=w2584, "padding value"=0.0, "matlab wave file"=path "2Pshutter", "DOtab"=0.0) -> (w2587:T18)
                                n372 = Build Array(w2587) -> (w2586:T17)
                                n373 = call "waveformparamsv2.vi"("command"="add DO", "add DO"=w2586) -> ()  [unwired: 3 in, 3 out]
                                }
                                frame 2 {
                                n374 = call "waveformparamsv2.vi"("command"="get") -> ("Params out"=w2599:T14)  [unwired: 4 in, 2 out]
                                n375 = in-place {
                                in-place-border: w2597 -> [w2603]
                                in-place-border: [w2602] -> w2596
                                n376 = in-place-cluster #7(w2599) -> ("DO parameters"=w2605:T17)
                                n377 = Delete From Array(array=w2605, length=1, index=w2603) -> (deleted portion=w2602:T17, array with subset deleted=w2604:T17)
                                n378 = in-place-cluster #7("DO parameters"=w2604) -> (w2598:T14)
                                }
                                n379 = call "waveformparamsv2.vi"("command"="set", "Params in"=w2598) -> ()  [unwired: 3 in, 3 out]
                                }
                                frame 3, Default {
                                }
                                frame 0 {
                                n380 = call "2pparameters.vi"("command"="get") -> ("params out"=w2612:T10)  [unwired: 1 in]
                                n381 = Unbundle By Name(w2612) -> ("wavdet"=w2609:bool, "autoshutter"=w2611:bool)
                                n382 = case shown="True" w2611 {
                                tunnel: w2610 -> [_ w2616]
                                tunnel: w2609 -> [_ w2615]
                                tunnel: [_ w2614] -> w2608
                                frame False {
                                }
                                frame True {
                                n383 = case shown="False" w2615 {
                                tunnel: w2616 -> [w2618 _]
                                tunnel: [w2617 _] -> w2614
                                frame False {
                                n384 = stacked-sequence {
                                tunnel: w2618 -> [w2620 w2634]
                                tunnel: [w2619 _] -> w2617
                                frame #0 {
                                n385 = call "waveformparamsv2.vi"("command"="get") -> ("Params out"=w2622:T14)  [unwired: 4 in, 2 out]
                                n386 = Unbundle By Name(w2622) -> ("DO parameters"=w2621:T17)
                                n387 = Index Array(array=w2621, index=w2620) -> (element=w2619:T18)
                                }
                                frame #1 {
                                w2633 = 0.0 ("padding value")
                                n388 = call "2pparameters.vi"("command"="get") -> ("params out"=w2631:T10)  [unwired: 1 in]
                                n389 = Unbundle By Name(w2631) -> ("srate"=w2628:sgl, "sAOxy"=w2630:i32)
                                n390 = To Double Precision Float(number=w2628) -> (double precision float=w2626:dbl)
                                n391 = To Double Precision Float(number=w2628) -> (double precision float=w2627:dbl)
                                n392 = To Double Precision Float(number=w2630) -> (double precision float=w2629:dbl)
                                n393 = Divide(x=w2627, y=w2629) -> (x/y=w2625:dbl)
                                n394 = call "replace DO wf param.vi"("Digital Freq (Hz)"=w2625, "Digital DC (%)"=100.0, "Digital phase"=w2633, "Sampling frequency (Hz)"=w2626, "Digital time offset (s)"=w2633, "index of DO wave"=w2634, "padding value"=w2633, "matlab wave file"=path "2Pshutter" ("matlab wave number")) -> ()  [unwired: 3 in]
                                }
                                }
                                }
                                frame True {
                                }
                                }
                                }
                                }
                                n395 = Build Array(w2608) -> (w2607:T17)
                                }
                                }
                              }
                              frame #7 {
                                n396 = Build Array(w2639, w2638) -> (w2641:bool[])
                                n397 = Boolean Array To Number(Boolean array=w2641) -> (number=w2640:u32)
                                n398 = case shown="2" w2640 {
                                tunnel: w2637 -> [_ w2683 _ w2690]
                                tunnel: [_ w2682 _ w2688] -> w2636
                                frame 1 {
                                n399 = call "2pparameters.vi"("command"="get") -> ("params out"=w2648:T10)  [unwired: 1 in]
                                n400 = Unbundle By Name(w2648) -> ("wavdet"=w2649:bool, "sAOxy"=w2651:i32, "refwfsize"=w2652:dbl, "srate Img"=w2650:sgl)
                                n401 = call "waveformsDObuffer.vi"("command"="get") -> ("DO wf out"=w2644:digitalwaveform[])  [unwired: 1 in]
                                n402 = case shown="False" w2649 {
                                tunnel: [w2657 w2667] -> w2646
                                tunnel: w2650 -> [w2662 w2678]
                                tunnel: w2651 -> [w2656 w2671]
                                tunnel: w2652 -> [_ w2675]
                                frame False {
                                w2660 = u16 0 items=["unsigned binary", "offset binary", "2's complement"] ("data format (offset binary)")
                                n403 = Initialize Array(sgl 1.0, w2656) -> (w2653:sgl[])
                                n404 = Reciprocal(x=w2662) -> (1/x=w2663:sgl)
                                n405 = Bundle By Name("Y"=w2653, "dt"=w2663) -> (w2658:waveform(sgl))  [unwired: 1 in]
                                n406 = call-poly <vilib>:"Analog to Digital.vi"("data format (offset binary)"=w2660, "compress digital (T)"=TRUE, "full-scale range (pk-pk)"=1.0, "resolution (16 bit)"=1, "analog waveform"=w2658) -> ("digital waveform"=w2657:digitalwaveform)  [unwired: 3 in, 3 out]
                                }
                                frame True {
                                w2670 = u16 0 items=["unsigned binary", "offset binary", "2's complement"] ("data format (offset binary)")
                                n407 = To Double Precision Float(number=w2671) -> (double precision float=w2676:dbl)
                                n408 = Initialize Array(sgl 1.0, w2671) -> (w2664:sgl[])
                                n409 = Divide(x=w2675, y=w2676) -> (x/y=w2673:dbl)
                                n410 = Round Toward +Infinity(x=w2673) -> (ceil(x): smallest int >= x=w2674:dbl)
                                n411 = for {
                                N: w2674 -> [_]
                                tunnel: w2664 -> [w2680]
                                tunnel: [w2680] -> w2677 mode=concatenating
                                }
                                n412 = Reciprocal(x=w2678) -> (1/x=w2679:sgl)
                                n413 = Bundle By Name("Y"=w2677, "dt"=w2679) -> (w2668:waveform(sgl))  [unwired: 1 in]
                                n414 = call-poly <vilib>:"Analog to Digital.vi"("data format (offset binary)"=w2670, "compress digital (T)"=TRUE, "full-scale range (pk-pk)"=1.0, "resolution (16 bit)"=1, "analog waveform"=w2668) -> ("digital waveform"=w2667:digitalwaveform)  [unwired: 3 in, 3 out]
                                }
                                }
                                n415 = Build Array (concatenate)(w2644, w2646) -> (w2642:digitalwaveform[])
                                n416 = call "waveformsDObuffer.vi"("DO wf in"=w2642, "command"="set") -> ()  [unwired: 1 out]
                                }
                                frame 2 {
                                n417 = call "waveformsDObuffer.vi"("command"="get") -> ("DO wf out"=w2685:digitalwaveform[])  [unwired: 1 in]
                                n418 = Delete From Array(array=w2685, length=1, index=w2683) -> (deleted portion=w2682:digitalwaveform[], array with subset deleted=w2681:digitalwaveform[])
                                n419 = call "waveformsDObuffer.vi"("DO wf in"=w2681, "command"="set") -> ()  [unwired: 1 out]
                                }
                                frame 3, Default {
                                }
                                frame 0 {
                                n420 = call "2pparameters.vi"("command"="get") -> ("params out"=w2692:T10)  [unwired: 1 in]
                                n421 = Unbundle By Name(w2692) -> ("autoshutter"=w2691:bool, "wavdet"=w2689:bool)
                                n422 = case shown="True" w2691 {
                                tunnel: w2690 -> [_ w2696]
                                tunnel: w2689 -> [_ w2695]
                                tunnel: [_ w2694] -> w2688
                                frame False {
                                }
                                frame True {
                                n423 = case shown="False" w2695 {
                                tunnel: w2696 -> [w2700 _]
                                tunnel: [w2698 _] -> w2694
                                frame False {
                                w2707 = u16 0 items=["unsigned binary", "offset binary", "2's complement"] ("data format (offset binary)")
                                n424 = call "2pparameters.vi"("command"="get") -> ("params out"=w2714:T10)  [unwired: 1 in]
                                n425 = Unbundle By Name(w2714) -> ("sAOxy"=w2716:i32, "srate Img"=w2715:sgl)
                                n426 = call "waveformsDObuffer.vi"("command"="get") -> ("DO wf out"=w2701:digitalwaveform[])  [unwired: 1 in]
                                n427 = Index Array(array=w2701, index=w2700) -> (element=w2699:digitalwaveform)
                                n428 = Build Array(w2699) -> (w2698:digitalwaveform[])
                                n429 = Initialize Array(sgl 1.0, w2716) -> (w2702:sgl[])
                                n430 = Reciprocal(x=w2715) -> (1/x=w2709:sgl)
                                n431 = Bundle By Name("Y"=w2702, "dt"=w2709) -> (w2705:waveform(sgl))  [unwired: 1 in]
                                n432 = call-poly <vilib>:"Analog to Digital.vi"("data format (offset binary)"=w2707, "compress digital (T)"=TRUE, "full-scale range (pk-pk)"=1.0, "resolution (16 bit)"=1, "analog waveform"=w2705) -> ("digital waveform"=w2712:digitalwaveform)  [unwired: 3 in, 3 out]
                                n433 = Replace Array Subset(array=w2701, new element=w2712, index=w2700) -> (w2697:digitalwaveform[])
                                n434 = call "waveformsDObuffer.vi"("DO wf in"=w2697, "command"="set") -> ()  [unwired: 1 out]
                                }
                                frame True {
                                }
                                }
                                }
                                }
                                }
                                }
                              }
                              frame #8 {
                                n435 = Build Array(w2720, w2719) -> (w2722:bool[])
                                n436 = Boolean Array To Number(Boolean array=w2722) -> (number=w2721:u32)
                                n437 = case shown="0" w2721 {
                                tunnel: w2718 -> [_ w2748 _ w2760]
                                tunnel: [_ w2747 _ w2758] -> w2717
                                frame 1 {
                                w2735 = 0.0 ("DOtab")
                                n438 = call "2pparameters.vi"("command"="get") -> ("params out"=w2733:T10)  [unwired: 1 in]
                                n439 = call "waveformparamsv2.vi"("command"="get") -> ("Params out"=w2743:T14)  [unwired: 4 in, 2 out]
                                n440 = Unbundle By Name(w2743) -> ("DO parameters"=w2741:T17)
                                n441 = Unbundle By Name(w2733) -> ("srate"=w2730:sgl, "sAOxy"=w2732:i32)
                                n442 = To Double Precision Float(number=w2730) -> (double precision float=w2728:dbl)
                                n443 = To Double Precision Float(number=w2730) -> (double precision float=w2729:dbl)
                                n444 = To Double Precision Float(number=w2732) -> (double precision float=w2724:dbl)
                                n445 = Divide(x=w2729, y=w2724) -> (x/y=w2731:dbl)
                                n446 = Index Array(array=w2741, index=0) -> (element=w2740:T18)
                                n447 = Divide(x=1.0 ("Digital DC (%)"), y=w2724) -> (x/y=w2726:dbl)
                                n448 = Multiply(x=100.0, y=w2726) -> (x*y=w2723:dbl)
                                n449 = Bundle By Name(cluster=w2740, "Digital DC (%)"=w2723, "Digital phase"=w2735, "Digital Freq (Hz)"=w2731, "Sampling frequency (Hz)"=w2728, "Digital time offset (s)"=w2735, "padding value"=0.0, "matlab wave file"=path "LT", "DOtab"=0.0) -> (w2738:T18)
                                n450 = Build Array(w2738) -> (w2737:T17)
                                n451 = call "waveformparamsv2.vi"("command"="add DO", "add DO"=w2737) -> ()  [unwired: 3 in, 3 out]
                                }
                                frame 2 {
                                n452 = call "waveformparamsv2.vi"("command"="get") -> ("Params out"=w2750:T14)  [unwired: 4 in, 2 out]
                                n453 = in-place {
                                in-place-border: w2748 -> [w2754]
                                in-place-border: [w2753] -> w2747
                                n454 = in-place-cluster #8(w2750) -> ("DO parameters"=w2756:T17)
                                n455 = Delete From Array(array=w2756, length=1, index=w2754) -> (deleted portion=w2753:T17, array with subset deleted=w2755:T17)
                                n456 = in-place-cluster #8("DO parameters"=w2755) -> (w2749:T14)
                                }
                                n457 = call "waveformparamsv2.vi"("command"="set", "Params in"=w2749) -> ()  [unwired: 3 in, 3 out]
                                }
                                frame 3, Default {
                                }
                                frame 0 {
                                n458 = local read "Measurement"() -> (w2762:T4)
                                n459 = To Unsigned Long Integer(number=w2762) -> (unsigned 32bit integer=w2761:u32)
                                n460 = case shown="5..7" w2761 {
                                tunnel: w2760 -> [_ w2764]
                                tunnel: [_ w2763] -> w2759
                                frame 0..4, Default {
                                }
                                frame 5..7 {
                                n461 = stacked-sequence {
                                tunnel: w2764 -> [w2766 w2775]
                                tunnel: [w2765 _] -> w2763
                                frame #0 {
                                n462 = call "waveformparamsv2.vi"("command"="get") -> ("Params out"=w2768:T14)  [unwired: 4 in, 2 out]
                                n463 = Unbundle By Name(w2768) -> ("DO parameters"=w2769:T17)
                                n464 = Index Array(array=w2769, index=w2766) -> (element=w2765:T18)
                                }
                                frame #1 {
                                w2783 = 0.0 ("padding value")
                                n465 = call "2pparameters.vi"("command"="get") -> ("params out"=w2781:T10)  [unwired: 1 in]
                                n466 = Unbundle By Name(w2781) -> ("srate"=w2779:sgl, "sAOxy"=w2780:i32)
                                n467 = To Double Precision Float(number=w2779) -> (double precision float=w2777:dbl)
                                n468 = To Double Precision Float(number=w2779) -> (double precision float=w2778:dbl)
                                n469 = To Double Precision Float(number=w2780) -> (double precision float=w2773:dbl)
                                n470 = Divide(x=1.0 ("Digital DC (%)"), y=w2773) -> (x/y=w2772:dbl)
                                n471 = Multiply(x=100.0, y=w2772) -> (x*y=w2771:dbl)
                                n472 = Divide(x=w2778, y=w2773) -> (x/y=w2776:dbl)
                                n473 = call "replace DO wf param.vi"("Digital Freq (Hz)"=w2776, "Digital DC (%)"=w2771, "Digital phase"=w2783, "Sampling frequency (Hz)"=w2777, "Digital time offset (s)"=w2783, "index of DO wave"=w2775, "padding value"=w2783, "matlab wave file"=path "LT" ("matlab wave number")) -> ()  [unwired: 3 in]
                                }
                                }
                                }
                                }
                                n474 = Build Array(w2759) -> (w2758:T17)
                                }
                                }
                              }
                              frame #9 {
                                n475 = Build Array(w2788, w2787) -> (w2790:bool[])
                                n476 = Boolean Array To Number(Boolean array=w2790) -> (number=w2789:u32)
                                n477 = case shown="2" w2789 {
                                tunnel: w2786 -> [_ w2842 _ w2846]
